vi "isDir.vi"(1 "path":path) -> (0 "is Dir?":bool)   [LabVIEW 2020]
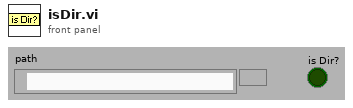
[diagram p1: front panel]
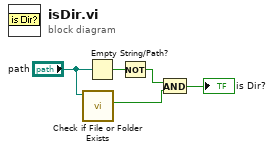
[diagram p0: block diagram]
diagram:
  n1 = call <vilib>:"Check if File or Folder Exists.vi"("path"="path") -> ("file or folder exists?"=w4:bool)  [unwired: 8 in, 2 out]
  n2 = Empty String/Path?(string/path="path") -> (empty?=w2:bool)
  n3 = Not(x=w2) -> (.not. x?=w5:bool)
  n4 = And(x=w5, y=w4) -> (x .and. y?=→"is Dir?":bool)
